vi "InitXnet.vi"(8 "error in (no error)":errorcluster, 10 "Measurement Signals":refnum<k21>[](array[refnum]), 11 "DAQList in":refnum<class "DAQList.lvclass">) -> (0 "error out":errorcluster, 3 "DAQList out":refnum<class "DAQList.lvclass">)   [LabVIEW 2019, in "XCP_DaqDtoId.lvlib" / "DAQList.lvclass"]
uses:
  DAQList.lvclass
  DAQList.lvclass/DAQList.ctl
  <vilib>/ECUMC/ECUMC.llb/MC StartStop Mode.ctt
  <vilib>/xnet/xnet.llb/XNET Create Session (Signal Input Waveform).vi
  TypeDef/Global.vi
  <vilib>/ECUMC/ECUMC.llb/MC Get Property.vi
  <vilib>/ECUMC/ECUMC.llb/MC Get Prop Meas Data Type.vi
  <vilib>/ECUMC/ECUMC.lvlib
  <resource>/objmgr/xnet.rc
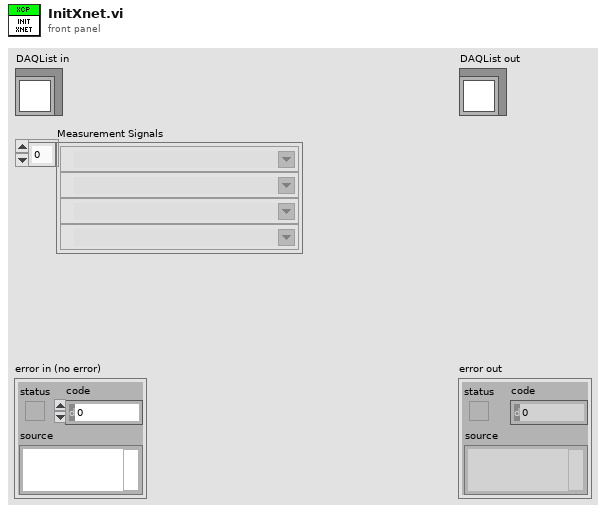
[diagram p1: front panel]
types:
  T1 = typedef "ECUMC.lvlib/MC StartStop Mode.ctt" = i32
  T2 = typedef "ECUMC.lvlib/MC Reference.ctt" = u32
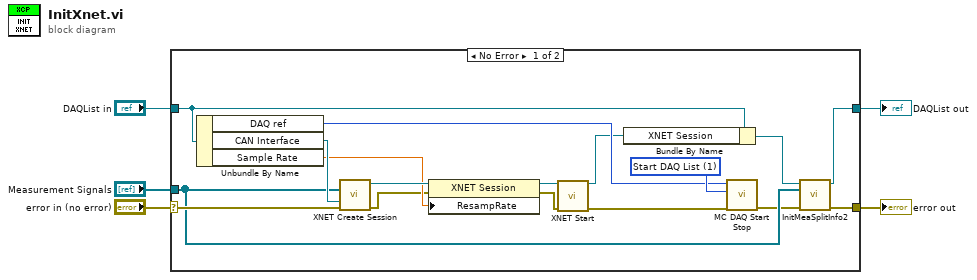
[diagram p0: block diagram]
diagram:
  n1 = case shown="No Error" "error in (no error)" {
    selector: "error in (no error)" -> [w21 w24]
    tunnel: [w13 w24] -> w4
    tunnel: [w14 w23] -> w2
    tunnel: "DAQList in" -> [w18 w23]
    tunnel: "Measurement Signals" -> [w16 _]
    frame No Error {
      w20 = T1 1 items=["Stop DAQ List", "Start DAQ List", "Transmit DAQ List to ECU", "Prepare For Start All", "Start All DAQ Lists", "Stop All DAQ Lists"] ("mode")
      n2 = Unbundle By Name(w18) -> ("DAQ ref"=w19:T2, "CAN Interface"=w22:refnum<k21>, "Sample Rate"=w9:dbl)
      n3 = call-poly <vilib>:"XNET Create Session.vi"("signal list"=w16, "interface"=w22, "error in (no error)"=w21) -> ("session out"=w10:refnum<k21>, "error out"=w8:errorcluster)  [unwired: 11 out]
      n4 = property class="XNET Session"(reference=w10, error in=w8, "ResampRate"=w9) -> (reference out=w7:refnum<k21>, error out=w6:errorcluster)
      n5 = call <vilib>:"XNET Start.vi"("session in"=w7, "error in (no error)"=w6) -> ("session out"=w11:refnum<k21>, "error out"=w12:errorcluster)  [unwired: 12 in]
      n6 = Bundle By Name(cluster=w18, "XNET Session"=w11) -> (w17:refnum<class "DAQList.lvclass">)
      n7 = call <vilib>:"MC DAQ Start Stop.vi"("error in"=w12, "mode"=w20, "DAQ ref in"=w19) -> ("error out"=w15:errorcluster)  [unwired: 7 in, 1 out]
      n8 = call "InitMeaSplitInfo2.vi"("error in (no error)"=w15, "Measurement Signals"=w16, "DAQList in"=w17) -> ("error out"=w13:errorcluster, "DAQList out"=w14:refnum<class "DAQList.lvclass">)  [unwired: 7 in]
    }
    frame Error {
    }
  }
  "error out" <- w4
  "DAQList out" <- w2
